vi "SendDashCAN.vi"   [LabVIEW 2015]
uses:
  <vilib>/RioEmbeddedCAN/RioEmbeddedCAN.llb/CANFrameControl.ctl
  NDashPage.ctl
  Global Data.vi
types:
  T1 = typedef "CANFrameControl.ctl" = cluster{"identifier":u32, "extended?":bool, "type":u8, "payload":u8[]}
  T2 = typedef "NDashPage.ctl" = enum16{"WaitingForCAN", "Driving", "LapTrigger", "Warning", "Systems", "Brakes", "Charging", "Suspension", "Drivetrain", "Performance"}
  T3 = typedef "FPGA Telemetry.ctl" = cluster{"CPU Load":cluster{"Total (%)":dbl, "Time Critical (%)":dbl, "Timed Structures (%)":dbl, "High (%)":dbl, "Above Normal (%)":dbl, "Normal (%)":dbl, "Background (%)":dbl, "Idle (%)":dbl, "ISR (%)":dbl}, "SVehicleStatus":cluster{"BMS Status":T4, "MC Status":T4, "Shutdown Status":T4, "sbRIO Status":T4, "Vehicle Status":T4, "Shutdown State":enum16{"NI.SC.Initial", "NI.SC.History", "NI.SC.ShallowHistory", "NI.SC.Terminal", "Coolant Pump Started/AIR's On", "AIRs On", "Precharge", "TSMS Off"}, "AIR Status":T7, "Remote Return to Pits":bool, "Reason for Shutdown":T8, "MC State Machine Status":enum16{"NI.SC.Initial", "NI.SC.History", "NI.SC.ShallowHistory", "NI.SC.Terminal", "Broadcast Diag", "Let Current Drop then Disable AIR's", "Enabled", "Disabled"}}, "iPhone HF Data":cluster{"gXiPhone":dbl, "gYiPhone":dbl, "gZiPhone":dbl, "nYawXiPhone":dbl, "nYawYiPhone":dbl, "nYawZiPhone":dbl}, "iPhone LF Data":cluster{"nLatiPhone":dbl, "nLongiPhone":dbl, "nGPSiPhone":dbl}, "stop":bool, "VSupplyOffset":fxp<+,12,4>, "VsbRIOSupply":fxp<+/-,25,6>, "bFPGALED":bool, "TSBRIO":fxp<+/-,33,17>, "rTPS2Unscaled":fxp<+/-,16,1>, "rTPS1Unscaled":fxp<+/-,16,1>, "bTPSConsistent":bool, "bTPSInRange":bool, "rThrottle":fxp<+/-,33,22>, "VTPS2":fxp<+/-,24,5>, "rTPS2":fxp<+/-,31,22>, "VTPS1":fxp<+/-,24,5>, "rTPS1":fxp<+/-,31,22>, "rTPS2Max":fxp<+,16,4>, "rTPS2Min":fxp<+,16,4>, "rTPS1Max":fxp<+,16,4>, "rTPS1Min":fxp<+,16,4>, "bCoolantPumpEnable":bool, "bRTDSEnable":bool, "bTSMSInStatus":bool, "bPosAIREnable":bool, "bBMSOK":bool, "bIMDOK":bool, "bBSPDOK":bool, "bSBRIOOK2":bool, "bSBRIOOK1":bool, "bTSMSOutStatus":bool, "eGreenDash":T9, "eYellowDash":T9, "eRedDash":T9, "bMotorControllerEnable":bool, "tCurrentLap":u32, "bNewLap":bool, "tLastLap":u32, "tLapMin":u32, "V5VSupply":fxp<+/-,24,5>, "bWheelRL":bool, "bWheelRR":bool, "bWheelFR":bool, "bWheelFL":bool, "VBrakePressureR":fxp<+/-,24,5>, "VBrakePressureF":fxp<+/-,24,5>, "bWheelRRStopped":bool, "bWheelRLStopped":bool, "bWheelFRStopped":bool, "bWheelFLStopped":bool, "tWheelRLPeriod":u32, "tWheelRRPeriod":u32, "tWheelFRPeriod":u32, "tWheelFLPeriod":u32, "bBrakeLight":bool, "VShockRR":fxp<+/-,24,5>, "VShockRL":fxp<+/-,24,5>, "VShockFR":fxp<+/-,24,5>, "VShockFL":fxp<+/-,24,5>, "IHighCurrent":fxp<+/-,24,15>, "ILowCurrent":fxp<+/-,24,15>, "pBrakeR":fxp<+,26,13>, "pBrakeF":fxp<+,26,13>, "bHighCurrentOK":bool, "bLowCurrentOK":bool, "bBrakeROK":bool, "bBrakeFOK":bool, "VSteerWheelMiddle":fxp<+/-,26,5>, "aSteerWheel":fxp<+/-,31,13>, "nWheelFL":fxp<+/-,32,16>, "nWheelFR":fxp<+/-,32,16>, "nWheelRL":fxp<+/-,32,16>, "nWheelRR":fxp<+/-,32,16>, "ADXL345 Output":T10, "Tire Diameter(m)":fxp<+,16,1>, "vWheelRR":fxp<+/-,32,18>, "vWheelRL":fxp<+/-,32,18>, "vWheelFR":fxp<+/-,32,18>, "vWheelFL":fxp<+/-,32,18>, "vWheelLowest":fxp<+/-,32,18>, "vWheelHighest":fxp<+/-,32,18>, "bAccel":bool, "vAxleF":fxp<+/-,33,19>, "vCar":fxp<+/-,33,19>, "sLap":fxp<+,32,12>, "rSlipRL":fxp<+/-,12,1>, "rSlipRR":fxp<+/-,12,1>, "rSlipFL":fxp<+/-,12,1>, "rSlipFR":fxp<+/-,12,1>, "NLap":u8, "tLapReference":u32, "tFastestLap":u32, "MTorqueRequest":dbl, "RS232 Error Out":cluster{"status":bool, "code":i32}}
  T4 = typedef "Subsystem Status.ctl" = cluster{"eStatusSeverity":T5, "NValue":sgl, "CMessage":T6, "bNotOK":bool}
  T5 = typedef "Subsystem Status Severity.ctl" = enum16{"Okay", "Short Warning", "Long Warning", "Return to Pits", "Error", "Danger"}
  T6 = typedef "Subsystem Status Message.ctl" = enum16{"ControllerTemperature", "MotorTemperature", "BatteryInternalResistance", "BatteryTemperature", "BatteryLowVoltage", "LVBattery", "sbRIOTemperature", "Precharge", "BSPD", "IMD", "RemoteReturnToPits", "EStopInterrupted", "NoCellComms", "MCOverSpeed", "MCOverCurrent", "MCOverVoltage", "MCInverterOverTemp", "MCDirectionCommand", "MCInverterTimeout", "MCDesatFault", "MCHWOverCurrent", "MCUnderVoltage", "MCCommandMessageLost", "MotorOverTemp", "MCModAOverTemp", "MCModBOverTemp", "MCModCOverTemp", "MCPCBOverTemp", "MCGateDrv1OverTemp", "MCDateDrv2OverTemp", "MCCurrentSensorFault", "MCResolverNotConnected", "ShutdownLatchTripped", "UnknownBMS", "RemoteEmergency"}
  T7 = typedef "AIR Status.ctl" = enum16{"Off", "Precharge", "On"}
  T8 = typedef "Reason for Shutdown.ctl" = enum16{"None", "BMS", "Shutdown", "sbRIO", "MC", "Remote"}
  T9 = typedef "Dash LED Status.ctl" = enum16{"Off", "Flashing", "On"}
  T10 = typedef "ADXL345 Output.ctl" = cluster{"X":fxp<+/-,14,4>, "Y":fxp<+/-,14,4>, "Z":fxp<+/-,14,4>}
  T11 = typedef "DashDriverInputs.ctl" = cluster{"ButtonsBitArray":u8, "NRedRotary":u8, "NYellowRotary":u8, "NBlackRotary":u8}
  T12 = typedef "CAN Message Queue.ctl" = refnum<k33>
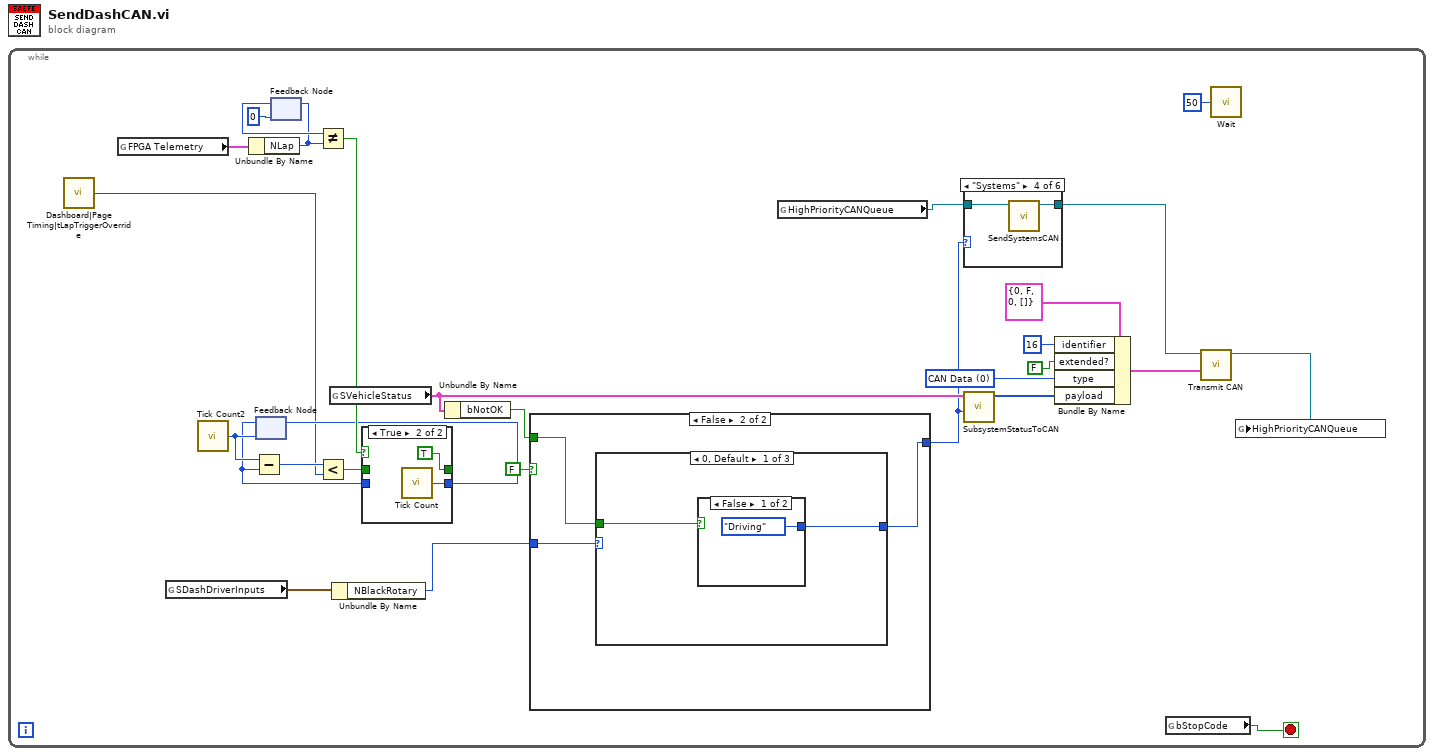
[diagram p0: block diagram]
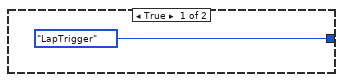
[diagram p3: hidden frame]
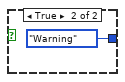
[diagram p4: hidden frame]
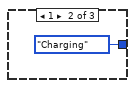
[diagram p5: hidden frame]
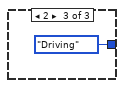
[diagram p6: hidden frame]
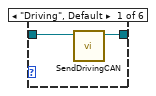
[diagram p7: hidden frame]
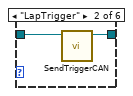
[diagram p8: hidden frame]
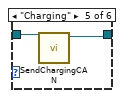
[diagram p10: hidden frame]
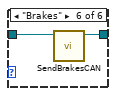
[diagram p11: hidden frame]
diagram:
  n1 = while {
    stop <- w3 stop-if-true
    w26 = u8 0 items=["CAN Data", "CAN Remote"] ("type")
    n2 = call "Dashboard|Page Timing|tLapTriggerOverride"() -> ("Value"=w11:u32)
    n3 = global read "Global Data.vi" "FPGA Telemetry"() -> (w20:T3)
    n4 = global read "Global Data.vi" "SDashDriverInputs"() -> (w8:T11)
    n5 = call "Tick Count2"() -> ("Tick Count(mSec)"=w14:u32)
    n6 = Unbundle By Name(w20) -> ("NLap"=w17:u8)
    n7 = feedback #1(w14) -> (w13:u32)
    n8 = Subtract(x=w14, y=w13) -> (x-y=w12:u32)
    n9 = feedback #2(u8 0 ("NLap")) -> (w18:u8)
    n10 = feedback-in #2(w17) -> ()
    n11 = Not Equal?(x=w18, y=w17) -> (x != y?=w16:bool)
    n12 = Less?(x=w12, y=w11) -> (x < y?=w10:bool)
    n13 = global read "Global Data.vi" "SVehicleStatus"() -> (w24:T4)
    n14 = Unbundle By Name(w8) -> ("NBlackRotary"=w7:u8)
    n15 = case shown="True" w16 {
      tunnel: [w29 TRUE] -> _
      tunnel: [w30 w31] -> w15
      tunnel: w13 -> [w30 _]
      tunnel: w10 -> [w29 _]
      frame False {
      }
      frame True {
        n16 = call "Tick Count"() -> ("Tick Count(mSec)"=w31:u32)
      }
    }
    n17 = feedback-in #1(w15) -> ()
    n18 = Unbundle By Name(w24) -> ("bNotOK"=w23:bool)
    n19 = case shown="False" FALSE {
      tunnel: w23 -> [_ w36]
      tunnel: [NDashPage."LapTrigger" ("NDashPage") w35] -> w21
      tunnel: w7 -> [_ w34]
      frame True {
      }
      frame False {
        n20 = case shown="0, Default" w34 {
          tunnel: w36 -> [w38 _ _]
          tunnel: [w37 NDashPage."Charging" ("NDashPage") NDashPage."Driving" ("NDashPage")] -> w35
          frame 0, Default {
            n21 = case shown="False" w38 {
              tunnel: [NDashPage."Driving" ("NDashPage") NDashPage."Warning" ("NDashPage")] -> w37
              frame False {
              }
              frame True {
              }
            }
          }
          frame 1 {
          }
          frame 2 {
          }
        }
      }
    }
    n22 = global read "Global Data.vi" "HighPriorityCANQueue"() -> (w4:T12)
    n23 = case shown="\"Systems\"" w21 {
      tunnel: [w43 w46 w47 w48 w50 w52] -> w5
      tunnel: w4 -> [w44 w45 w47 w49 w51 w53]
      frame "Driving", Default {
        n24 = call "SendDrivingCAN.vi"("CANTXQueueIn"=w44) -> ("CANTXQueueOut"=w43:T12)  [unwired: 10 in]
      }
      frame "LapTrigger" {
        n25 = call "SendTriggerCAN.vi"("CANTXQueueIn"=w45) -> ("CANTXQueueOut"=w46:T12)  [unwired: 10 in]
      }
      frame "Warning" {
      }
      frame "Systems" {
        n26 = call "SendSystemsCAN.vi"("CANTXQueueIn"=w49) -> ("CANTXQueueOut"=w48:T12)  [unwired: 10 in]
      }
      frame "Charging" {
        n27 = call "SendChargingCAN.vi"("CANTXQueueIn"=w51) -> ("CANTXQueueOut"=w50:T12)  [unwired: 10 in]
      }
      frame "Brakes" {
        n28 = call "SendBrakesCAN.vi"("CANTXQueueIn"=w53) -> ("CANTXQueueOut"=w52:T12)  [unwired: 10 in]
      }
    }
    n29 = call "SubsystemStatusToCAN.vi"("NDashPage"=w21, "Subystem Status"=w24) -> ("Array"=w25:u8[])  [unwired: 9 in]
    n30 = Bundle By Name(cluster=T1 {"identifier"=0, "extended?"=FALSE, "type"=0, "payload"=[]} ("CAN frame"), "identifier"=u32 16, "extended?"=FALSE, "type"=w26, "payload"=w25) -> (w6:T1)
    n31 = global read "Global Data.vi" "bStopCode"() -> (w3:bool)
    n32 = call "Transmit CAN.vi"("CAN Queue"=w5, "CAN frame"=w6) -> ("CAN Queue Out"=w1:T12)  [unwired: 8 in]
    n33 = call "Wait"("Count(mSec)"=u32 50) -> ()  [unwired: 1 out]
    n34 = global write "Global Data.vi" "HighPriorityCANQueue"(w1) -> ()
  }
